vi "Table Select Section Cut to 1D Array.vi"(11 "Table Ref In":refnum<vi>) -> (1 "Cut Value":string[](array[string]), 3 "Table Ref Out":refnum<vi>)   [LabVIEW 2024]
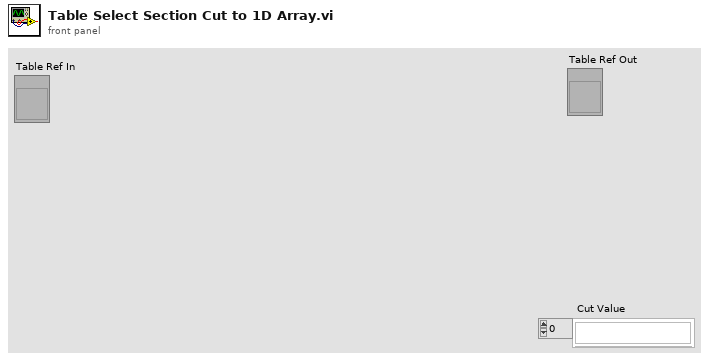
[diagram p1: front panel]
types:
  T1 = typedef "LVRowAndColumnTypeDef.ctl" = cluster{"Row":i32, "Column":i32}
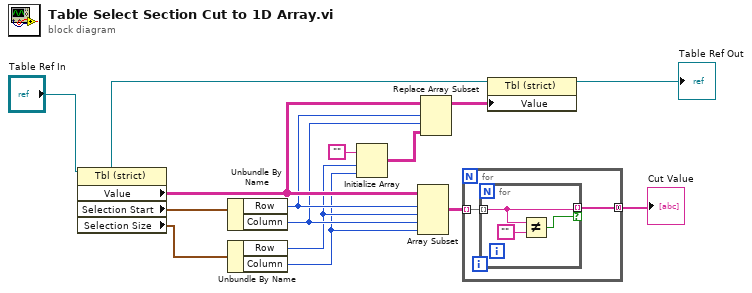
[diagram p0: block diagram]
diagram:
  n1 = property class="Tbl (strict)"(reference="Table Ref In") -> (reference out=w12:refnum<vi>, "Value"=w8:string[][], "Selection Start"=w14:T1, "Selection Size"=w13:T1)  [unwired: 1 in, 1 out]
  n2 = Unbundle By Name(w14) -> ("Row"=w7:i32, "Column"=w3:i32)
  n3 = Unbundle By Name(w13) -> ("Row"=w2:i32, "Column"=w1:i32)
  n4 = Initialize Array("", w2, w1) -> (w5:string[][])
  n5 = Array Subset(array=w8, index (row)=w7, length (row)=w2, index (col)=w3, length (col)=w1) -> (w10:string[][])
  n6 = Replace Array Subset(array=w8, new element=w5, index (row)=w7, index (col)=w3) -> (w4:string[][])
  n7 = for {
    tunnel: w10 -> [w17] mode=indexing
    tunnel: [w16] -> w9 mode=concatenating
    n8 = for {
      tunnel: [w18] -> w16 mode=indexing if=w19
      tunnel: w17 -> [w18] mode=indexing
      n9 = Not Equal?(x=w18, y="") -> (x != y?=w19:bool)
    }
  }
  "Cut Value" <- w9
  n10 = property class="Tbl (strict)"(reference=w12, "Value"=w4) -> (reference out=→"Table Ref Out":refnum<vi>)  [unwired: 1 in, 1 out]
